vi "PAQmem_get_one_layer_UnsavedRAM.vi"(8 "error in (no error)":errorcluster, 11 "PAQ-memory in":refnum<class "PAQ-memory.lvclass">) -> (0 "error out":errorcluster, 1 "Data2save":T1, 2 "TableName":string, 3 "PAQ-memory out":refnum<class "PAQ-memory.lvclass">)   [LabVIEW 2020, in "PAQ-memory.lvclass"]
doc: "Get the latest unsaved RAM from one layer of PAQ data"
uses:
  PAQ-memory.lvclass
  PAQ-memory.lvclass/PAQ-memory.ctl
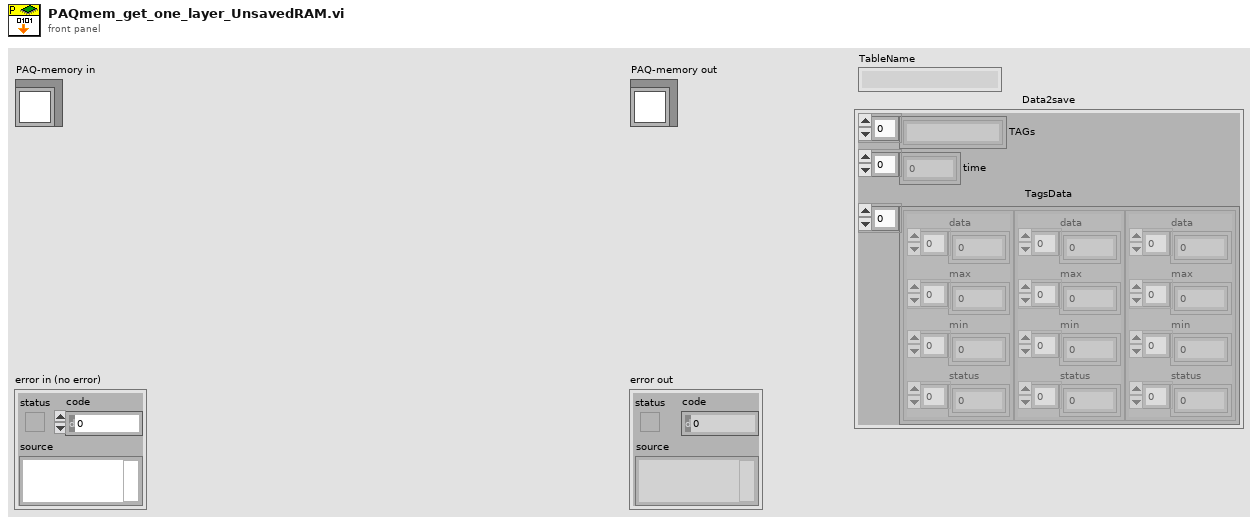
[diagram p1: front panel]
types:
  T1 = cluster{"TAGs":string[], "time":dbl[], "TagsData":cluster{"data":dbl[], "max":dbl[], "min":dbl[], "status":u32[]}[]}
  T2 = cluster{"data":dbl[], "max":dbl[], "min":dbl[], "status":u32[]}[]
  T3 = cluster{"data":dbl[], "max":dbl[], "min":dbl[], "status":u32[]}
  T4 = cluster{"TAGindex":i32, "Location":i32, "Size":i32}
  T5 = typedef "FAMM.lvclass/typedef_PAQdata.ctl" = cluster{"TAGs":string[], "Time":refnum<data-value>, "TAGdata":cluster{"source":refnum<data-value>, "status":refnum<data-value>, "data":refnum<data-value>, "max":refnum<data-value>, "min":refnum<data-value>}[]}
  T6 = cluster{"time":dbl[], "data":dbl[], "max":dbl[], "min":dbl[], "status":u32[]}
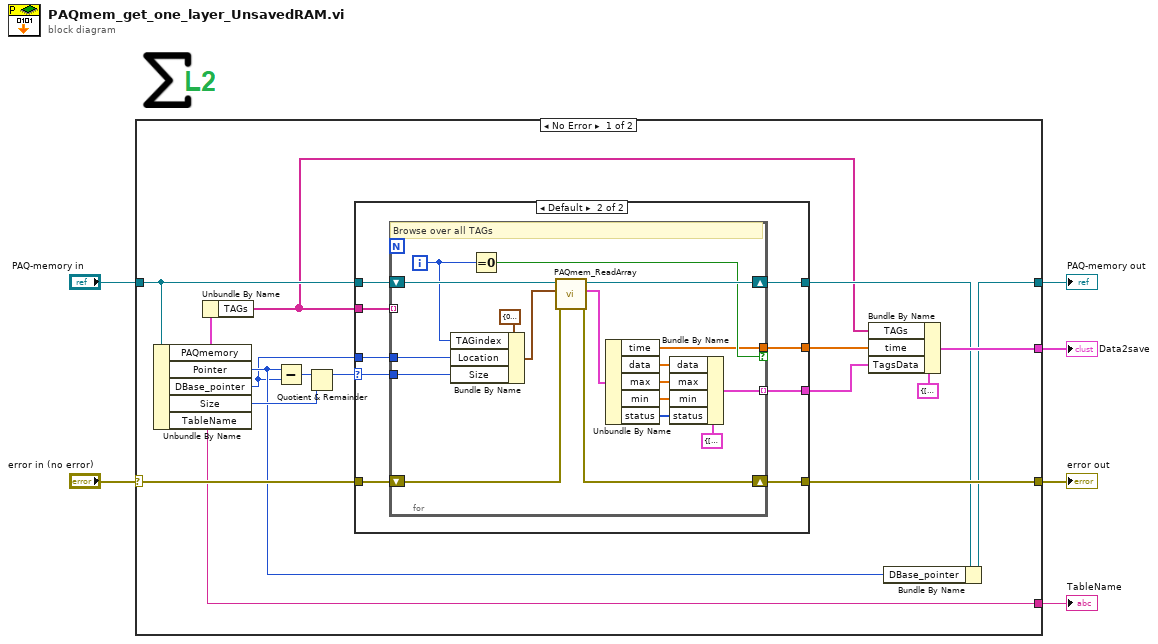
[diagram p0: block diagram]
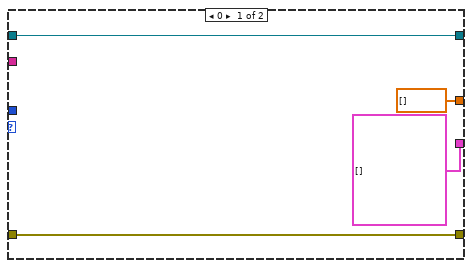
[diagram p2: hidden frame]
diagram:
  n1 = case shown="No Error" "error in (no error)" {
    selector: "error in (no error)" -> [w22 w56]
    tunnel: [w17 w56] -> w5
    tunnel: [w14 w55] -> w3
    tunnel: "PAQ-memory in" -> [w23 w55]
    tunnel: [w18 _] -> w2
    tunnel: [w7 _] -> w1
    frame No Error {
      n2 = Unbundle By Name(w23) -> ("PAQmemory"=w13:T5, "Pointer"=w9:i32, "DBase_pointer"=w8:i32, "Size"=w10:i32, "TableName"=w7:string)
      n3 = Unbundle By Name(w13) -> ("TAGs"=w12:string[])
      n4 = Subtract(x=w9, y=w8) -> (x-y=w16:i32)
      n5 = Quotient & Remainder(x=w16, y=w10) -> (x-y*floor(x/y)=w11:i32)  [unwired: 1 out]
      n6 = case shown="Default" w11 {
        selector: w11 -> [_ w28]
        tunnel: w23 -> [w27 w36]
        tunnel: w22 -> [w24 w35]
        tunnel: [T2 [] w34] -> w20
        tunnel: [dbl[] [] ("time") w33] -> w19
        tunnel: [w24 w32] -> w17
        tunnel: w8 -> [_ w31]
        tunnel: [w27 w30] -> w15
        tunnel: w12 -> [_ w29]
        frame 0 {
        }
        frame Default {
          n7 = for {
            shift-right: [w53] -> w30
            shift-left: w36 -> [w54]
            shift-right: [w50] -> w32
            shift-left: w35 -> [w51]
            tunnel: [w43] -> w34 mode=indexing
            tunnel: [w37] -> w33 if=w42
            tunnel: w28 -> [w41]
            tunnel: w31 -> [w40]
            tunnel: w29 -> [_] mode=indexing
            i -> [w38]
            # "Browse over all TAGs"
            n8 = Bundle By Name(cluster=T4 {"TAGindex"=0, "Location"=0, "Size"=0} ("ChunkDefinition"), "TAGindex"=w38, "Location"=w40, "Size"=w41) -> (w39:T4)
            n9 = Equal To 0?(x=w38) -> (x = 0?=w42:bool)
            n10 = call "PAQmem_ReadArray.vi"("error in (no error)"=w51, "ChunkDefinition"=w39, "PAQ-memory in"=w54) -> ("error out"=w50:errorcluster, "OneTagData"=w49:T6, "PAQ-memory out"=w53:refnum<class "PAQ-memory.lvclass">)  [unwired: 6 in]
            n11 = Unbundle By Name(w49) -> ("time"=w37:dbl[], "data"=w44:dbl[], "max"=w45:dbl[], "min"=w46:dbl[], "status"=w47:u32[])
            n12 = Bundle By Name(cluster=T3 {"data"=[], "max"=[], "min"=[], "status"=[]} ("OneTagData"), "data"=w44, "max"=w45, "min"=w46, "status"=w47) -> (w43:T3)
          }
        }
      }
      n13 = Bundle By Name(cluster=T1 {"TAGs"=[], "time"=[], "TagsData"=[]} ("Data2save"), "TAGs"=w12, "time"=w19, "TagsData"=w20) -> (w18:T1)
      n14 = Bundle By Name(cluster=w15, "DBase_pointer"=w9) -> (w14:refnum<class "PAQ-memory.lvclass">)
    }
    frame Error {
    }
  }
  "error out" <- w5
  "PAQ-memory out" <- w3
  "Data2save" <- w2
  "TableName" <- w1
